vi "Get Auto Range Value [ARV] Core.vi"(8 "error in (no error)":errorcluster, 11 "IVI_DMM in":refnum<class "IVI_DMM.lvclass">) -> (0 "error out":errorcluster, 2 "actual range":dbl format="%^.2e", 3 "IVI_DMM out":refnum<class "IVI_DMM.lvclass">)   [LabVIEW 2013, in "IVI_DMM.lvlib" / "IVI_DMM.lvclass"]
doc: "This VI returns the actual range the DMM is currently using, even while it is auto-ranging.\n\nNote: \n\n(1) This VI is part of the IviDmmAutoRangeValue [ARV] extension group."
uses:
  IVI_DMM.lvclass
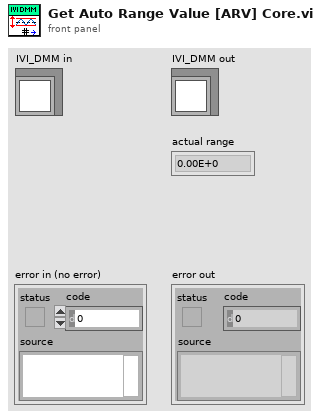
[diagram p1: front panel]
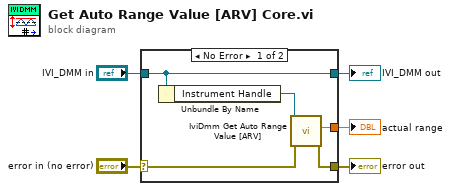
[diagram p0: block diagram]
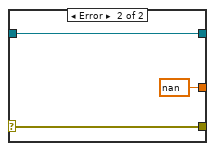
[diagram p2: hidden frame]
diagram:
  n1 = case shown="No Error" "error in (no error)" {
    selector: "error in (no error)" -> [w8 w13]
    tunnel: [w7 w13] -> w4
    tunnel: [w10 w12] -> w2
    tunnel: "IVI_DMM in" -> [w10 w12]
    tunnel: [w6 nan ("actual range")] -> w1
    frame No Error {
      n2 = Unbundle By Name(w10) -> ("Instrument Handle"=w9:refnum<k15>)
      n3 = call <vilib>:"IviDmm Get Auto Range Value [ARV].vi"("error in (no error)"=w8, "instrument handle"=w9) -> ("error out"=w7:errorcluster, "actual range"=w6:dbl)  [unwired: 7 in, 1 out]
    }
    frame Error {
    }
  }
  "error out" <- w4
  "IVI_DMM out" <- w2
  "actual range" <- w1
